vi "Top-Level Launcher.vi"() -> ()   [LabVIEW 2014]
uses:
  Build/Build Links Application.vi
  Links Application/LinksApplication.lvclass
panel:
  in  "Rebuild":bool
  in  "LaunchEXE":bool
  in  "File to Analyze":path caption="Select a LabVIEW File (VI, LVClass, LVLib) to analyze its static linkages"
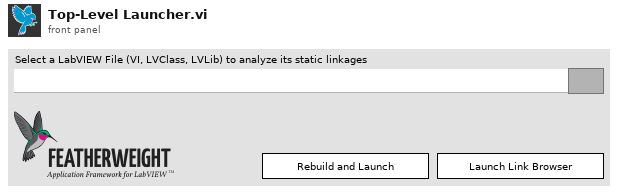
[diagram p1: front panel]
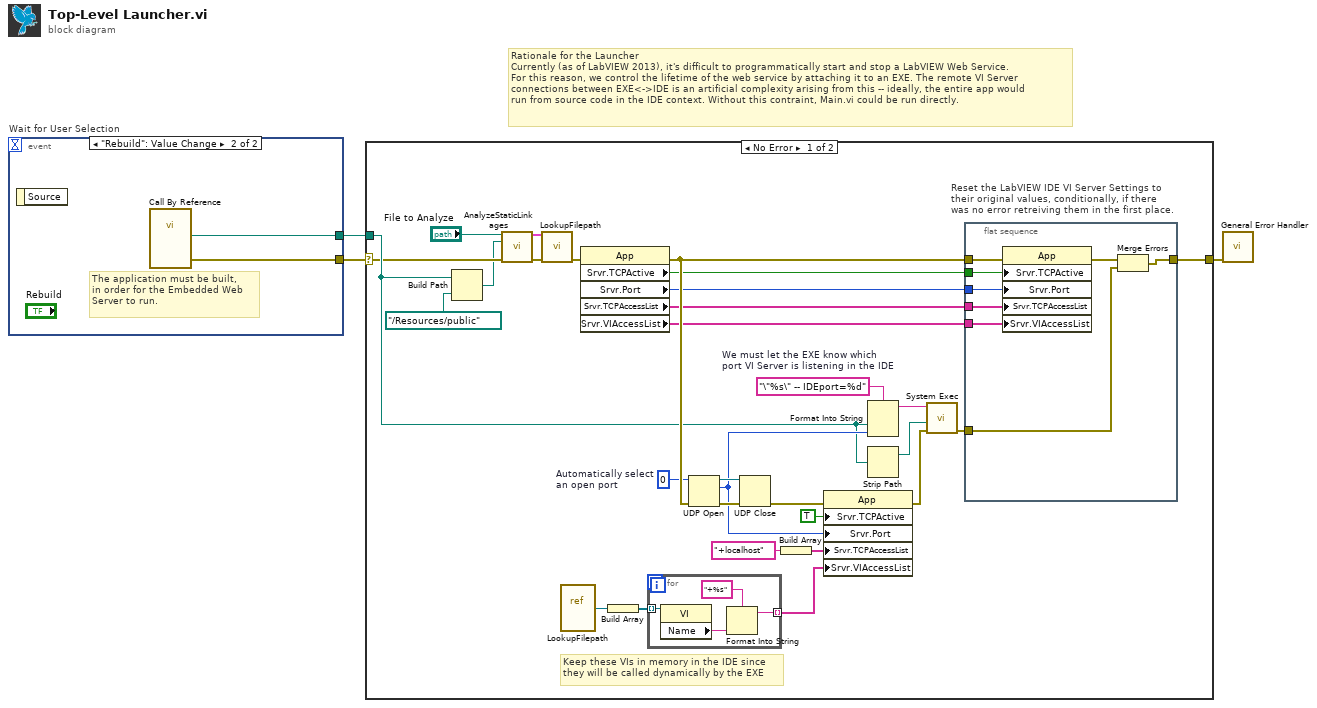
[diagram p0: block diagram]
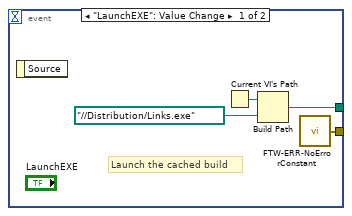
[diagram p2: hidden frame]
diagram:
  # "Rationale for the Launcher\nCurrently (as of LabVIEW 2013), it's difficult to programmatically start and stop a LabVIEW Web Service.\nFor this reason, we control the lifetime of the web service by attaching it to an EXE. The remote VI Server\nconnections between EXE<->IDE is an artificial complexity arising from this -- ideally, the entire app would\nrun from source code in the IDE context. Without this contraint, Main.vi could be run directly."
  n1 = event "Wait for User Selection" shown="[1] \"Rebuild\": Value Change" {
    selector: _ -> [_ _]
    dyn-events: _ -> [_ _]
    timeout: _ -> [_ _]
    tunnel: [w7 w8] -> w2
    tunnel: [w4 w9] -> w1
    event "LaunchEXE": Value Change {
      # "Launch the cached build"
      n2 = event-data() -> ()  [unwired: 1 in, 1 out]
      n3 = Current VI's Path() -> (path=w6:path)
      n4 = Build Path(base path=w6, name or relative path=path "../../Distribution/Links.exe") -> (appended path=w4:path)
      n5 = call "FTW-ERR-NoErrorConstant.vi"() -> ("no error"=w7:errorcluster)
    }
    event "Rebuild": Value Change {
      # "The application must be built,\nin order for the Embedded Web\nServer to run."
      n6 = event-data() -> ()  [unwired: 1 in, 1 out]
      n7 = call-by-ref "?"() -> ("error out"=w8:errorcluster, "Path to Application"=w9:path)  [unwired: 12 in, 2 out]
    }
  }
  n8 = case shown="No Error" w2 {
    selector: w2 -> [w14 w52]
    tunnel: w1 -> [w16 _]
    tunnel: [w39 w52] -> w3
    frame No Error {
      w23 = u16 0  # Automatically select an open port
      w37 = "\"%s\" -- IDEport=%d"  # We must let the EXE know which port VI Server is listening in the IDE
      # "Keep these VIs in memory in the IDE since\nthey will be called dynamically by the EXE"
      n9 = Build Path(base path=w16, name or relative path=path "../Resources/public") -> (appended path=w13:path)
      n10 = call "AnalyzeStaticLinkages.vi"("LabVIEW File to Analyze"="File to Analyze", "Public Server Directory"=w13, "error in"=w14) -> ("Filepath Map"=w11:cluster{"Key":string, "Filepath":path}[], "error out"=w12:errorcluster)  [unwired: 11 in]
      n11 = call "LookupFilepath.vi"("Filepath Map"=w11, "error in"=w12) -> ("error out"=w10:errorcluster)  [unwired: 13 in]
      n12 = vi-ref "LookupFilepath.vi"() -> (w21:refnum<vi>)
      n13 = property class="App"(error in=w10) -> (error out=w32:errorcluster, "Srvr.TCPActive"=w30:bool, "Srvr.Port"=w29:u32, "Srvr.TCPAccessList"=w28:string[], "Srvr.VIAccessList"=w26:string[])  [unwired: 1 in, 1 out]
      n14 = Build Array(w21) -> (w20:refnum<vi>[])
      n15 = for {
        tunnel: w20 -> [w41] mode=indexing
        tunnel: [w40] -> w19 mode=indexing
        n16 = property class="VI"(reference=w41) -> ("Name"=w42:string)  [unwired: 1 in, 2 out]
        n17 = Format Into String(format string="+%s", w42) -> (resulting string=w40:string)  [unwired: 2 in, 1 out]
      }
      n18 = UDP Open(8:w32, 11:w23) -> (port=w22:refnum<k16>, 0:w34:errorcluster, 2:w18:u16)  [unwired: 3 in]
      n19 = UDP Close(connection ID=w22, 8:w34) -> (error out=w35:errorcluster)  [unwired: 1 out]
      n20 = Build Array("+localhost") -> (w25:string[])
      n21 = property class="App"(error in=w35, "Srvr.TCPActive"=TRUE ("Server:TCP Listener Active"), "Srvr.Port"=w18, "Srvr.TCPAccessList"=w25, "Srvr.VIAccessList"=w19) -> (error out=w31:errorcluster)  [unwired: 1 in, 1 out]
      n22 = Format Into String(format string=w37, w16, w18) -> (resulting string=w36:string)  [unwired: 2 in, 1 out]
      n23 = Strip Path(path=w16) -> (stripped path=w38:path)  [unwired: 1 out]
      n24 = call <vilib>:"System Exec.vi"("error in (no error)"=w31, "working directory"=w38, "command line"=w36) -> ("error out"=w27:errorcluster)  [unwired: 5 in, 3 out]
      n25 = flat-sequence "Reset the LabVIEW IDE VI Server Settings to\ntheir original values, conditionally, if there\nwas no error retreiving them in the first place." {
        tunnel: w32 -> [w51]
        tunnel: w30 -> [w50]
        tunnel: w29 -> [w49]
        tunnel: w28 -> [w48]
        tunnel: [w45] -> w39
        tunnel: w27 -> [w46]
        tunnel: w26 -> [w44]
        frame #0 {
          n26 = property class="App"(error in=w51, "Srvr.TCPActive"=w50, "Srvr.Port"=w49, "Srvr.TCPAccessList"=w48, "Srvr.VIAccessList"=w44) -> (error out=w47:errorcluster)  [unwired: 1 in, 1 out]
          n27 = Merge Errors(w47, w46) -> (w45:errorcluster)
        }
      }
    }
    frame Error {
    }
  }
  n28 = call <vilib>:"General Error Handler.vi"("error in (no error)"=w3) -> ()  [unwired: 10 in, 5 out]
